vi "uTTA_GetSamplingSettings.vi"(8 "error in":errorcluster, 11 "VISA Refnum in":refnum<visa-resource-name>) -> (0 "error out":errorcluster, 1 "Fast SampleRate":i32, 2 "Low SampleRate":dbl, 3 "VISA Refnum out":refnum<visa-resource-name>, 4 "Fast Prescaler":dbl, 5 "Max. Multiplier":i32, 7 "Received":string)   [LabVIEW 2021]
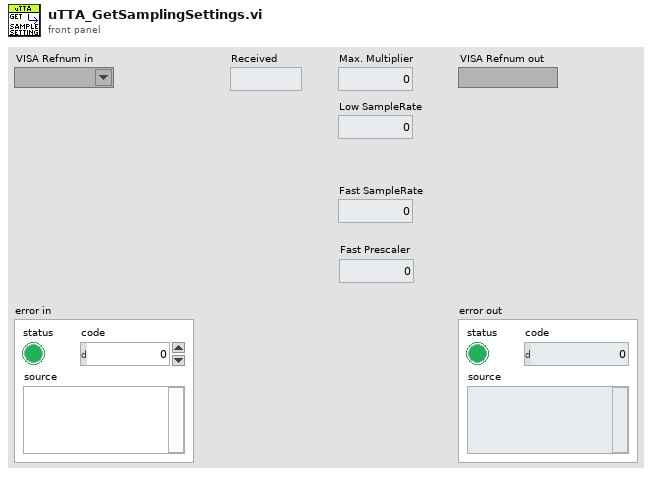
[diagram p1: front panel]
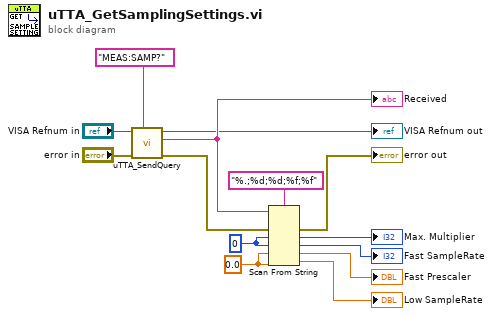
[diagram p0: block diagram]
diagram:
  w10 = 0.0 ("default value 1")
  w9 = 0 ("default value 1")
  n1 = call "uTTA_SendQuery.vi"("Send String"="MEAS:SAMP?" ("format string"), "error in (no error)"="error in", "VISA Refnum in"="VISA Refnum in") -> ("error out"=w7:errorcluster, "Received"=w5:string, "VISA Refnum out"=→"VISA Refnum out":refnum<visa-resource-name>)  [unwired: 6 in]
  "Received" <- w5
  n2 = Scan From String(format string="%.;%d;%d;%f;%f", input string=w5, error in=w7, default 1=w9, default 2=w9, default 3=w10, default 4=w10) -> (error out=→"error out":errorcluster, output 1=→"Max. Multiplier":i32, output 2=→"Fast SampleRate":i32, output 3=→"Fast Prescaler":dbl, output 4=→"Low SampleRate":dbl)  [unwired: 1 in, 2 out]
